vi "Pre Launch Init.vi"(11 "PublishingViewable In":refnum<class "PublishingViewable.lvclass">) -> (0 "error out":errorcluster, 3 "PublishingViewable Out":refnum<class "PublishingViewable.lvclass">)   [LabVIEW 2017, in "TestPubSubRouting.lvlib" / "PublishingViewable.lvclass"]
doc: "(<B>Filename</B>: Actor Framework.lvlib:Actor.lvclass:Pre Launch Init.vi)\n\nDefines behavior that occurs after the Launch Nested Actor method is invoked but before the actor's Actor Core method begins running.\n\nBy default, this method does nothing. A descendant class may override it to define behavior."
uses:
  PublishingViewable.lvclass
  Source/Framework/IViewable/IViewable/IViewable.lvclass
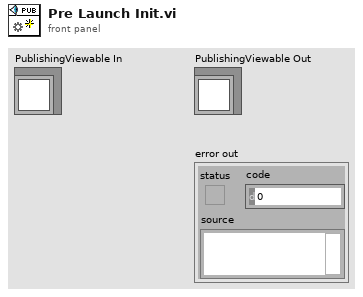
[diagram p1: front panel]
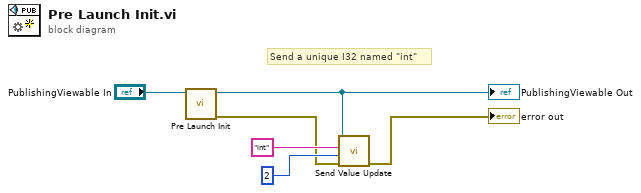
[diagram p0: block diagram]
diagram:
  # "Send a unique I32 named \"int\""
  n1 = call-parent "Pre Launch Init.vi"("IViewable in"="PublishingViewable In") -> ("error out"=w2:errorcluster, "IViewable out"=w5:refnum<class "PublishingViewable.lvclass">)  [unwired: 9 in]
  "PublishingViewable Out" <- w5
  n2 = call-dynamic "Send Value Update.vi"("error in (no error)"=w2, "Value"=2, "Datum Name"="int", "IViewable in"=w5) -> ("error out"=→"error out":errorcluster)  [unwired: 7 in]
